vi "IHM Git.vi"() -> ()   [LabVIEW 2021]
panel:
  in  "Exit":bool
  in  "Commande onglets":enum32{"Page 1"}(tab)
  in  "Push":bool
  in  "Chemin":path
  in  "Message":string
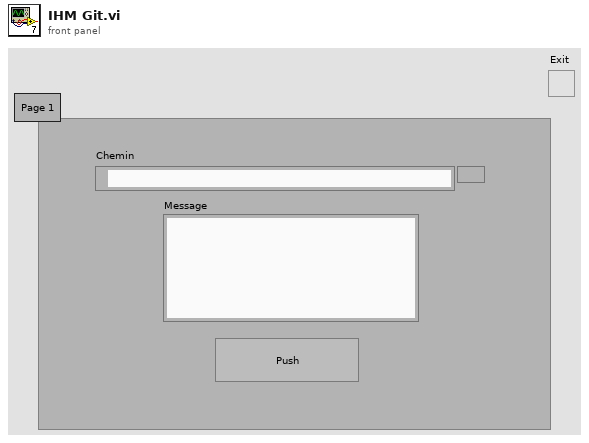
[diagram p1: front panel]
types:
  T1 = enum32{"invalid app kind", "Development System", "Run Time System", "Student Edition", "Embedded LabVIEW", "Evaluation", "Custom"}
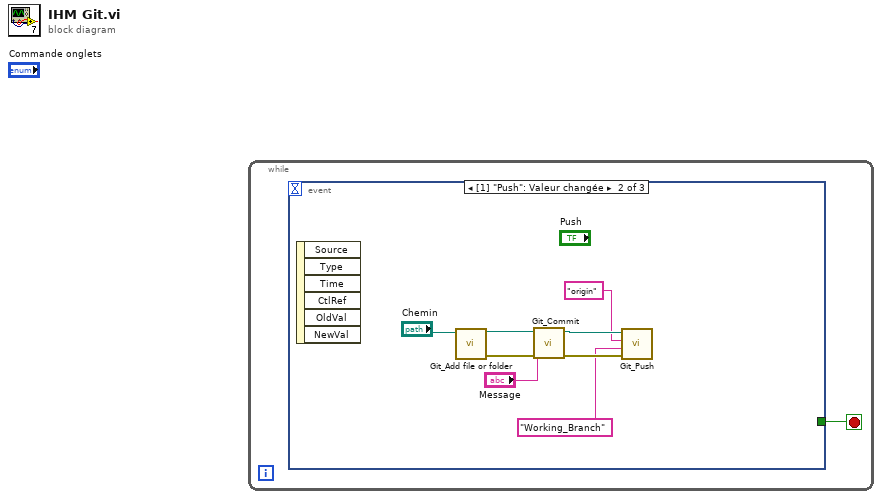
[diagram p0: block diagram]
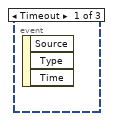
[diagram p2: hidden frame]
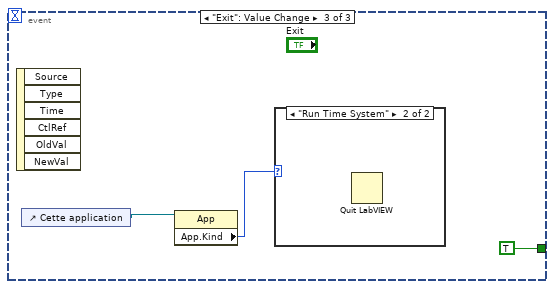
[diagram p3: hidden frame]
diagram:
  n1 = while {
    stop <- w1 stop-if-true
    n2 = event shown="[1] \"Push\": Valeur changée" {
      selector: _ -> [_ _ _]
      dyn-events: _ -> [_ _ _]
      timeout: _ -> [_ _ _]
      tunnel: [_ _ TRUE] -> w1
      event Timeout {
        n3 = event-data() -> ()  [unwired: 1 in, 3 out]
      }
      event "Push": Value Change {
        n4 = event-data() -> ()  [unwired: 1 in, 6 out]
        n5 = call "Git_Add file or folder.vi"("Chemin in"="Chemin") -> ("error out"=w7:errorcluster, "Chemin out"=w8:path)  [unwired: 9 in]
        n6 = call "Git_Commit.vi"("error in (no error)"=w7, "Message"="Message", "Chemin in"=w8) -> ("error out"=w5:errorcluster, "Chemin out"=w4:path)  [unwired: 7 in]
        n7 = call "Git_Push.vi"("error in (no error)"=w5, "Branch Name"="Working_Branch", "Remote Name"="origin", "Chemin in"=w4) -> ()  [unwired: 6 in, 2 out]
      }
      event "Exit": Value Change {
        n8 = event-data() -> ()  [unwired: 1 in, 6 out]
        n9 = control-ref of="Cette application"() -> (w11:refnum<vi>)
        n10 = property class="App"(reference=w11) -> ("App.Kind"=w12:T1)  [unwired: 1 in, 2 out]
        n11 = case shown="\"Run Time System\"" w12 {
          frame "invalid app kind", Default {
          }
          frame "Run Time System" {
            n12 = Quit LabVIEW() -> ()  [unwired: 1 in]
          }
        }
      }
    }
  }
